vi "RunCaraya.vi"   [LabVIEW 2013]
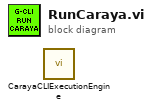
[diagram p0: block diagram]
diagram:
  n1 = call "CarayaCLIExecutionEngine.vi"() -> ()  [unwired: 12 in]
